vi "OPO_read_points.vi"(3 "error in (no error)":errorcluster, 5 "file path (dialog if empty)":path) -> (0 "error out":errorcluster, 1 "Delay List":string[][](array[string]), 2 "Cancelled?":bool)   [LabVIEW 2019]
doc: "Reads in a delay list"
uses:
  <vilib>/Utility/file.llb/Read Delimited Spreadsheet (string).vi
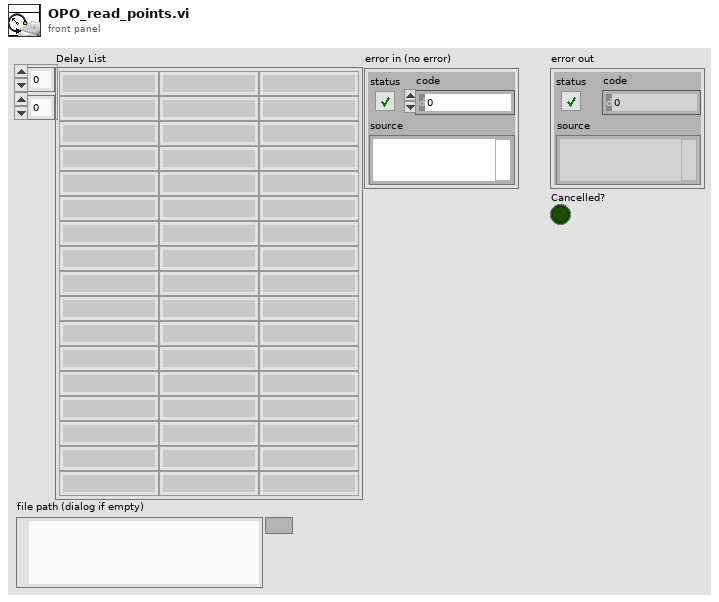
[diagram p1: front panel]
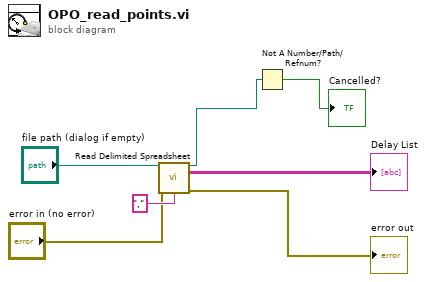
[diagram p0: block diagram]
diagram:
  n1 = call-poly <vilib>:"Read Delimited Spreadsheet.vi"("file path (dialog if empty)"="file path (dialog if empty)", "error in (no error)"="error in (no error)", "delimiter (\\t)"="," ("delimiter (\\t)")) -> ("new file path (Not A Path if cancelled)"=w2:path, "all rows"=→"Delay List":string[][], "error out"=→"error out":errorcluster)  [unwired: 7 in, 3 out]
  n2 = Not A Number/Path/Refnum?(number/path/refnum=w2) -> (NaN/Path/Refnum?=→"Cancelled?":bool)
